vi "Send Error to Sytem Log.vi"(8 "error in (no error)":errorcluster, 9 "Error to Send":errorcluster, 10 "Error Title or Message":string) -> (0 "error out":errorcluster)   [LabVIEW 2018, in "Error Handler.lvlib"]
uses:
  Error Handler.lvlib
  Testing UI 1/Testing UI 1.lvlib
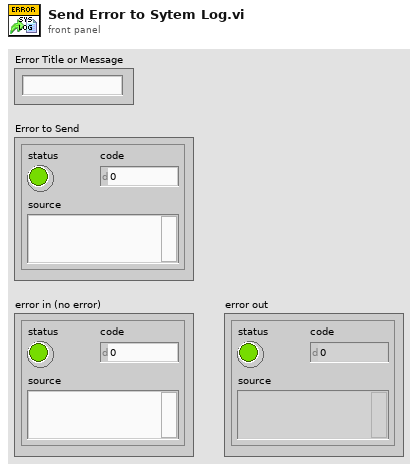
[diagram p1: front panel]
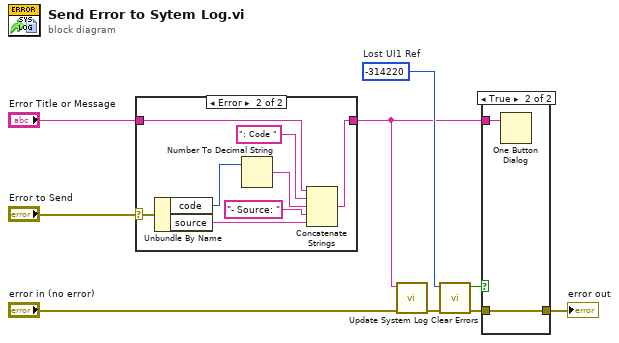
[diagram p0: block diagram]
diagram:
  w5 = -314220  # Lost UI1 Ref
  n1 = case shown="Error" "Error to Send" {
    selector: "Error to Send" -> [_ w13]
    tunnel: [w10 w18] -> w1
    tunnel: "Error Title or Message" -> [w10 w15]
    frame No Error {
    }
    frame Error {
      n2 = Unbundle By Name(w13) -> ("code"=w14:i32, "source"=w11:string)
      n3 = Number To Decimal String(number=w14) -> (decimal integer string=w17:string)  [unwired: 1 in]
      n4 = Concatenate Strings(w15, ": Code " ("string"), w17, "- Source: " ("string"), w11) -> (w18:string)
    }
  }
  n5 = call "Update System Log.vi"("error in"="error in (no error)", "Message"=w1) -> ("error out"=w6:errorcluster)  [unwired: 9 in]
  n6 = call <vilib>:"Clear Errors.vi"("error in (no error)"=w6, "specific error code to clear (0: all)"=w5) -> ("error out"=w2:errorcluster, "specific error cleared?"=w4:bool)  [unwired: 4 in]
  n7 = case shown="True" w4 {
    tunnel: [w19 w21] -> w3
    tunnel: w2 -> [w19 w21]
    tunnel: w1 -> [_ w20]
    frame False {
    }
    frame True {
      n8 = One Button Dialog(message=w20) -> ()  [unwired: 1 in, 1 out]
    }
  }
  "error out" <- w3
